vi "outcomesorter.vi"(8 "Outcome Total elecFee":dbl[](array[numeric]), 11 "OUTCOME":T1(array[cluster])) -> (3 "sorted Outcome":T1(array[cluster]))   [LabVIEW 2014]
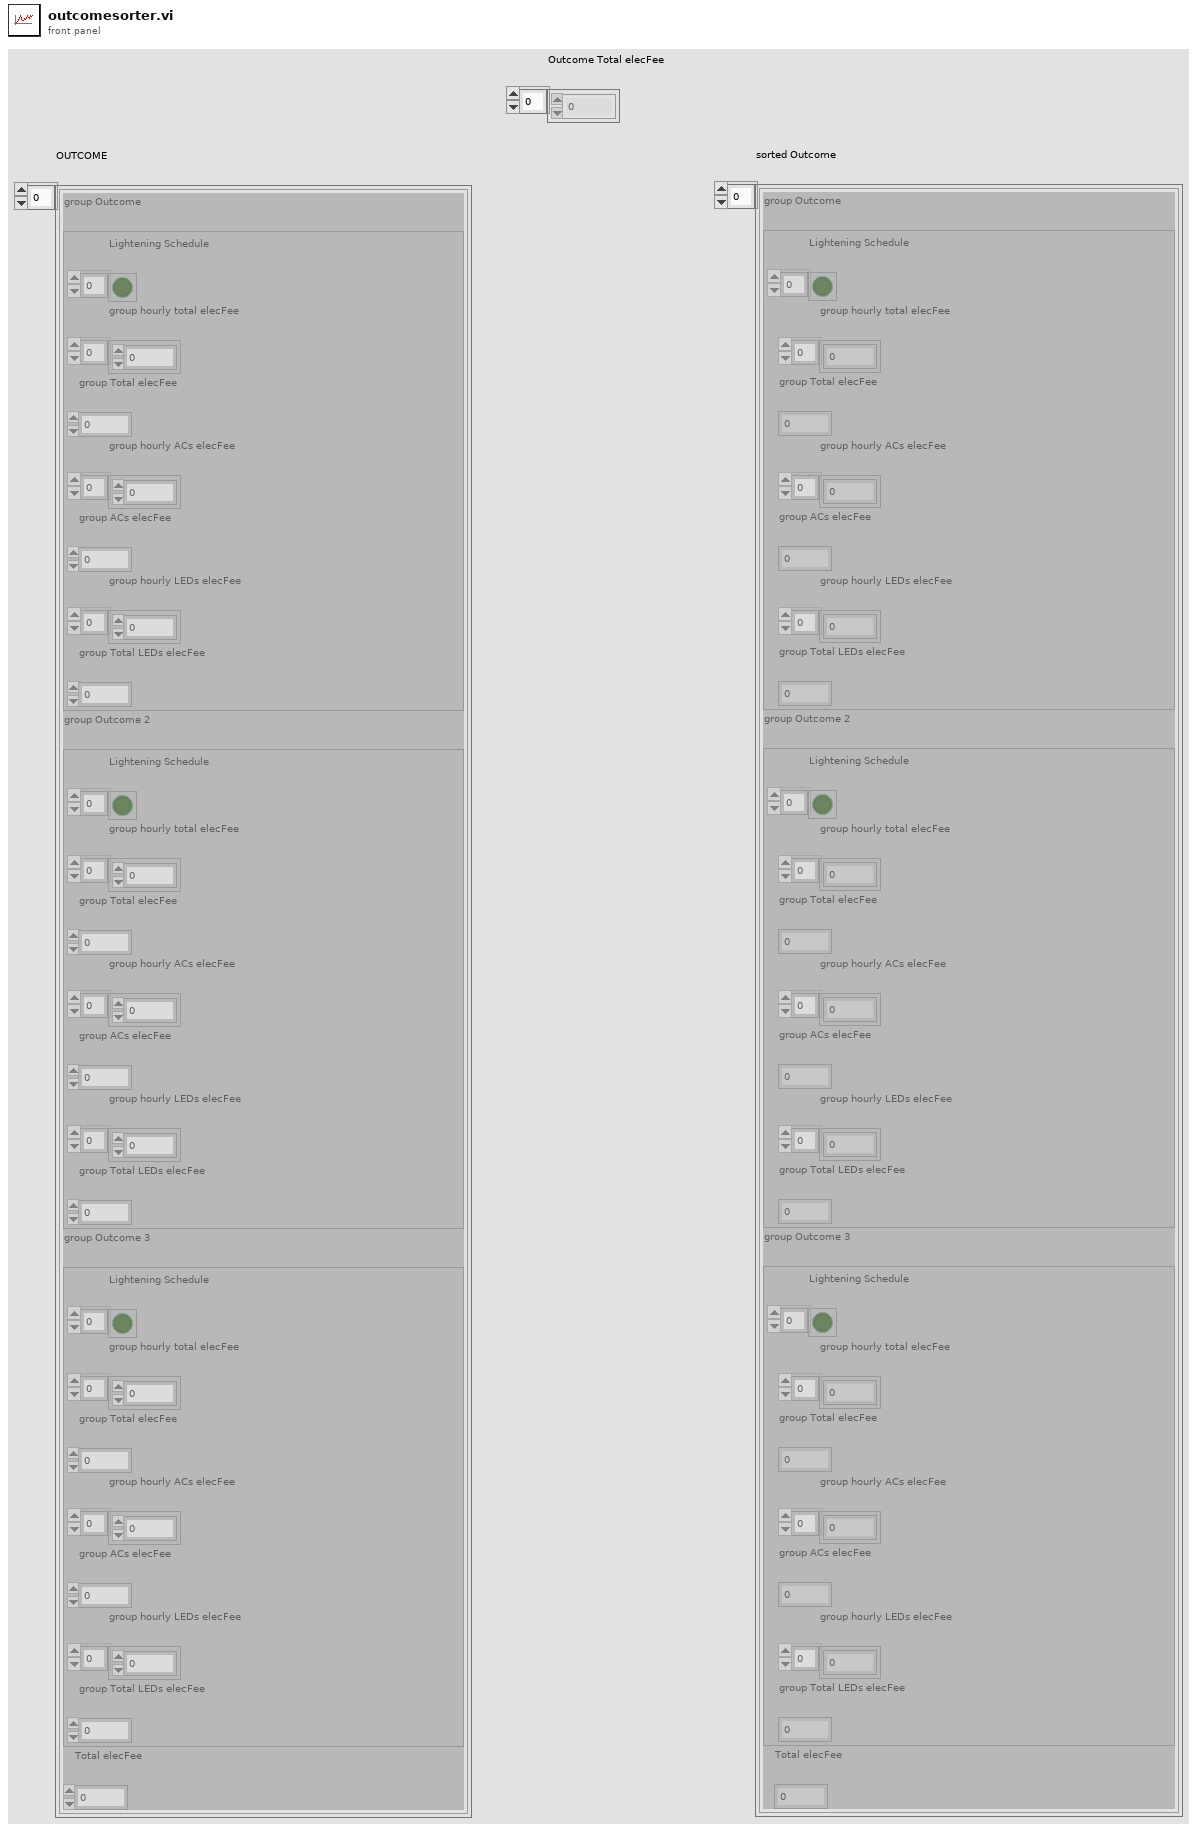
[diagram p1: front panel]
types:
  T1 = cluster{"group Outcome":cluster{"Lightening Schedule":bool[], "group hourly total elecFee":dbl[], "group Total elecFee":dbl, "group hourly ACs elecFee":dbl[], "group ACs elecFee":dbl, "group hourly LEDs elecFee":dbl[], "group Total LEDs elecFee":dbl}, "group Outcome 2":cluster{"Lightening Schedule":bool[], "group hourly total elecFee":dbl[], "group Total elecFee":dbl, "group hourly ACs elecFee":dbl[], "group ACs elecFee":dbl, "group hourly LEDs elecFee":dbl[], "group Total LEDs elecFee":dbl}, "group Outcome 3":cluster{"Lightening Schedule":bool[], "group hourly total elecFee":dbl[], "group Total elecFee":dbl, "group hourly ACs elecFee":dbl[], "group ACs elecFee":dbl, "group hourly LEDs elecFee":dbl[], "group Total LEDs elecFee":dbl}, "Total elecFee":dbl}[]
  T2 = cluster{"group Outcome":cluster{"Lightening Schedule":bool[], "group hourly total elecFee":dbl[], "group Total elecFee":dbl, "group hourly ACs elecFee":dbl[], "group ACs elecFee":dbl, "group hourly LEDs elecFee":dbl[], "group Total LEDs elecFee":dbl}, "group Outcome 2":cluster{"Lightening Schedule":bool[], "group hourly total elecFee":dbl[], "group Total elecFee":dbl, "group hourly ACs elecFee":dbl[], "group ACs elecFee":dbl, "group hourly LEDs elecFee":dbl[], "group Total LEDs elecFee":dbl}, "group Outcome 3":cluster{"Lightening Schedule":bool[], "group hourly total elecFee":dbl[], "group Total elecFee":dbl, "group hourly ACs elecFee":dbl[], "group ACs elecFee":dbl, "group hourly LEDs elecFee":dbl[], "group Total LEDs elecFee":dbl}, "Total elecFee":dbl}
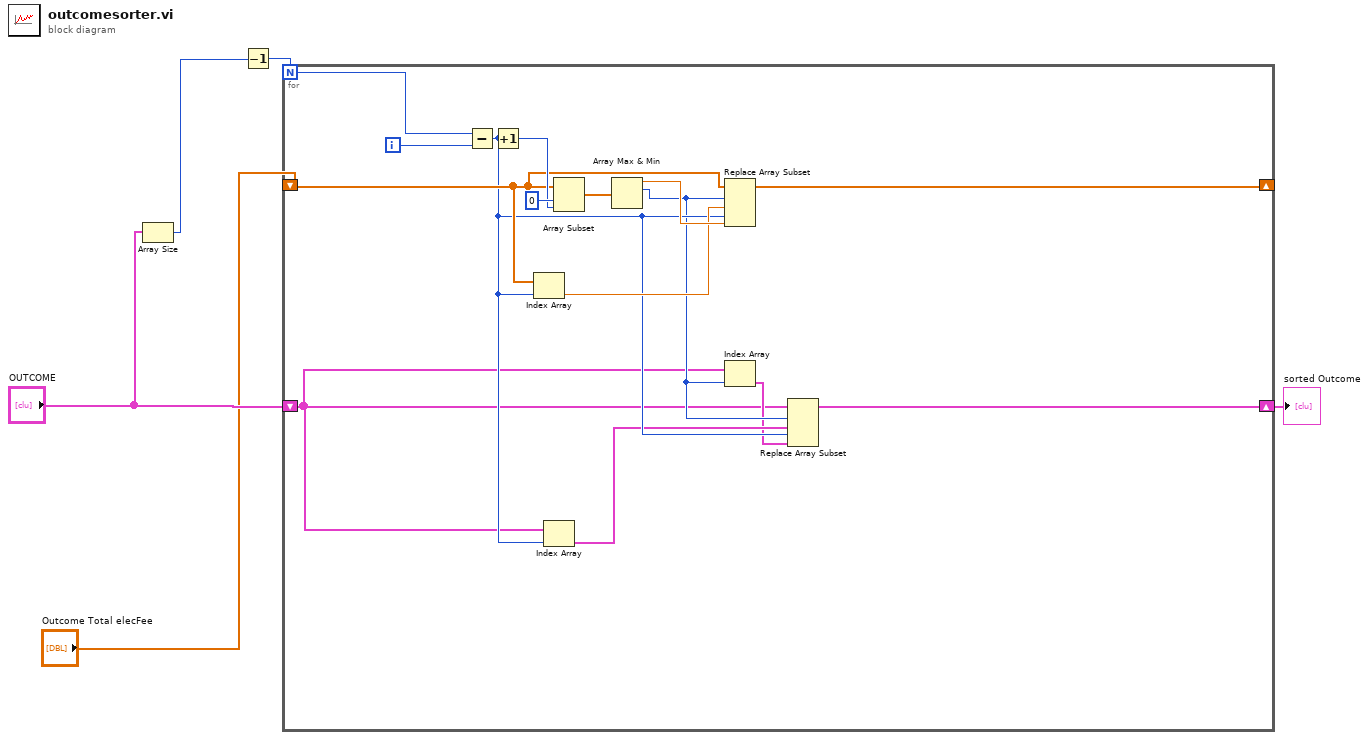
[diagram p0: block diagram]
diagram:
  n1 = Array Size(array="OUTCOME") -> (size(s)=w5:i32)
  n2 = Decrement(x=w5) -> (x-1=w4:i32)
  n3 = for {
    N: w4 -> [w14]
    shift-right: [w6] -> w1
    shift-left: "OUTCOME" -> [w7]
    shift-right: [w12] -> _
    shift-left: "Outcome Total elecFee" -> [w13]
    i -> [w15]
    n4 = Subtract(x=w14, y=w15) -> (x-y=w11:i32)
    n5 = Increment(x=w11) -> (x+1=w17:i32)
    n6 = Index Array(array=w13, index=w11) -> (element=w16:dbl)
    n7 = Index Array(array=w7, index=w11) -> (element=w10:T2)
    n8 = Array Subset(array=w13, index=0, length=w17) -> (w19:dbl[])
    n9 = Array Max & Min(array=w19) -> (max value=w18:dbl, max index (indices)=w9:i32)  [unwired: 2 out]
    n10 = Replace Array Subset(array=w13, new element #1=w16, index #1=w9, new element #2=w18, index #2=w11) -> (w12:dbl[])
    n11 = Index Array(array=w7, index=w9) -> (element=w8:T2)
    n12 = Replace Array Subset(array=w7, new element #1=w10, index #1=w9, new element #2=w8, index #2=w11) -> (w6:T1)
  }
  "sorted Outcome" <- w1
